vi "Servo PWM.vi"(1 "Drive Pin":refnum<k21>, 2 "Duty Cycle":u32) -> ()   [LabVIEW 2019]
uses:
  <vilib>/rvi/eio/common/nirviEmuTemplateMethod_errors.vi
  <vilib>/eio/EIONode/EIONode.xnode
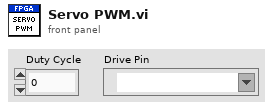
[diagram p1: front panel]
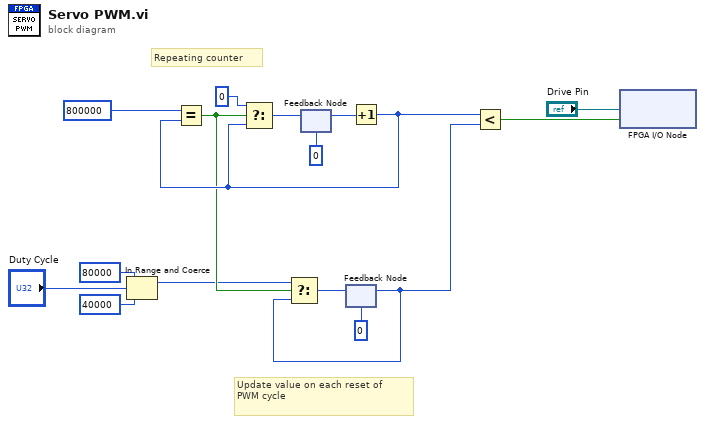
[diagram p0: block diagram]
diagram:
  # "Repeating counter"
  # "Update value on each reset of \nPWM cycle"
  n1 = In Range and Coerce(upper limit=u32 80000, x="Duty Cycle", lower limit=u32 40000) -> (coerced(x)=w2:u32)  [unwired: 1 out]
  n2 = feedback #1(u32 0 ("Compare Value")) -> (w11:u32)
  n3 = feedback #2(u32 0 ("Compare Value")) -> (w7:u32)
  n4 = Increment(x=w11) -> (x+1=w8:u32)
  n5 = Equal?(x=u32 800000 ("Period"), y=w8) -> (x = y?=w6:bool)
  n6 = Select(t=u32 0, s=w6, f=w8) -> (s? t:f=w13:u32)
  n7 = Select(t=w2, s=w6, f=w7) -> (s? t:f=w14:u32)
  n8 = feedback-in #1(w13) -> ()
  n9 = feedback-in #2(w14) -> ()
  n10 = Less?(x=w8, y=w7) -> (x < y?=w5:bool)
  n11 = xnode "FPGA I/O Node"("I/O项"=w5, "FPGA I/O输入"="Drive Pin") -> ()  [unwired: 1 out]
